vi "ziExample-Boxcar.vi"() -> ()   [LabVIEW 2009]
doc: "Control a Zurich instrument device via the LabOne Labview API. \nRequirements: Zurich Instruments UHFLI \nThis example retrives boxcar samples from a Zurich Instruments UHFLI instrument.\n\n© Zurich Instruments AG, www.zhinst.com"
uses:
  <instrlib>/Zurich Instruments LabOne/Public/Configure/ziSetValueDoubleArray.vi
  <instrlib>/Zurich Instruments LabOne/Public/Utility/ziTicksToS_single.vi
  <instrlib>/Zurich Instruments LabOne/Public/Configure/ziSetValueDouble.vi
  <instrlib>/Zurich Instruments LabOne/Public/Utility/ziTicksToS_vector.vi
  <instrlib>/Zurich Instruments LabOne/Public/Data/ziGetEventDoubleDataTS.vi
  <instrlib>/Zurich Instruments LabOne/Public/Data/ziGetEventPWAWave.vi
  <instrlib>/Zurich Instruments LabOne/Public/Data/ziGetEventIntDataTS.vi
  <instrlib>/Zurich Instruments LabOne/Zurich Instruments LabOne.lvlib
  <vilib>/Analysis/NI_AALBase.lvlib
panel:
  in  "boxcars/0/periods":dbl=1.0 caption="Boxcar Periods"
  in  "boxcars/0/windowsize":dbl=3e-09 caption="Window Size"
  in  "boxcars/0/windowstart":dbl=75.0 caption="Window Start"
  out "boxcarstd":dbl caption="Boxcar STD" format="%e"
  out "boxcaravg":dbl caption="Boxcar AVG" format="%e"
  out "periods":dbl caption="Periods" format="%0.2f"
  out "All Values (V) 2":cluster{"Timestamp(s)":dbl[], "Value":dbl[]}(graph)
  out "Error Out":errorcluster
  in  "Address":string="DEV"
  out "Selected Device":string
  out "Update Rate (1/s)":dbl(graph)
  out "All Values (V)":cluster{"Timestamp(s)":dbl[], "Value":dbl[]}(graph)
  in  "stop":bool
  # "ziExample-Boxcar.vi\nRequirements: UHFLI\nsee block diagram for VI description"
  # "Tested Devices:\n- UHFLI"
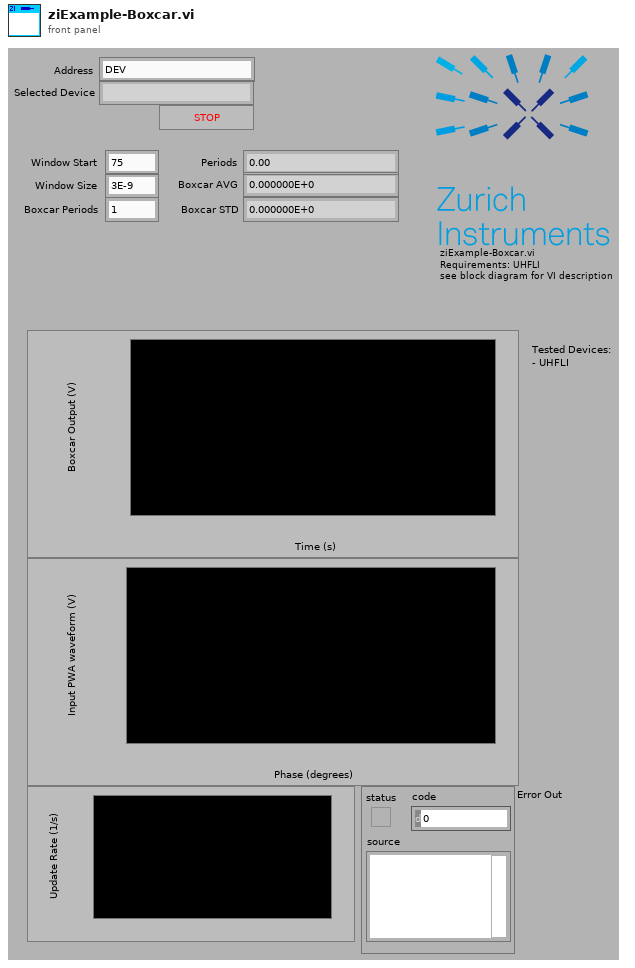
[diagram p1: front panel]
types:
  T1 = typedef "Zurich Instruments LabOne.lvlib/ziTypeHandle.ctl" = cluster{"handleValid":bool, "Conn":u64, "Path Prefix":string, "Handle":u64, "Connected":bool, "Clockbase(s)":dbl}
  T2 = typedef "Zurich Instruments LabOne.lvlib/ziTypeDoubleDataTS.ctl" = cluster{"Timestamp (ticks)":u64[], "Value":dbl[]}
  T3 = typedef "Zurich Instruments LabOne.lvlib/ziTypePWAWave.ctl" = cluster{"Timestamp (ticks)":u64, "SampleCount":u64, "InputSelect":i32, "OscSelect":i32, "Harmonic":i32, "BinCount":i32, "Frequency (Hz)":dbl, "PWAType":u8, "Mode":u8, "Overflow":u8, "Commensurable":u8, "BinPhase":dbl[], "X":dbl[], "Y":dbl[], "countBin":u32[]}
  T4 = typedef "Zurich Instruments LabOne.lvlib/ziTypeIntegerDataTS.ctl" = cluster{"Timestamp (ticks)":u64[], "Value":i64[]}
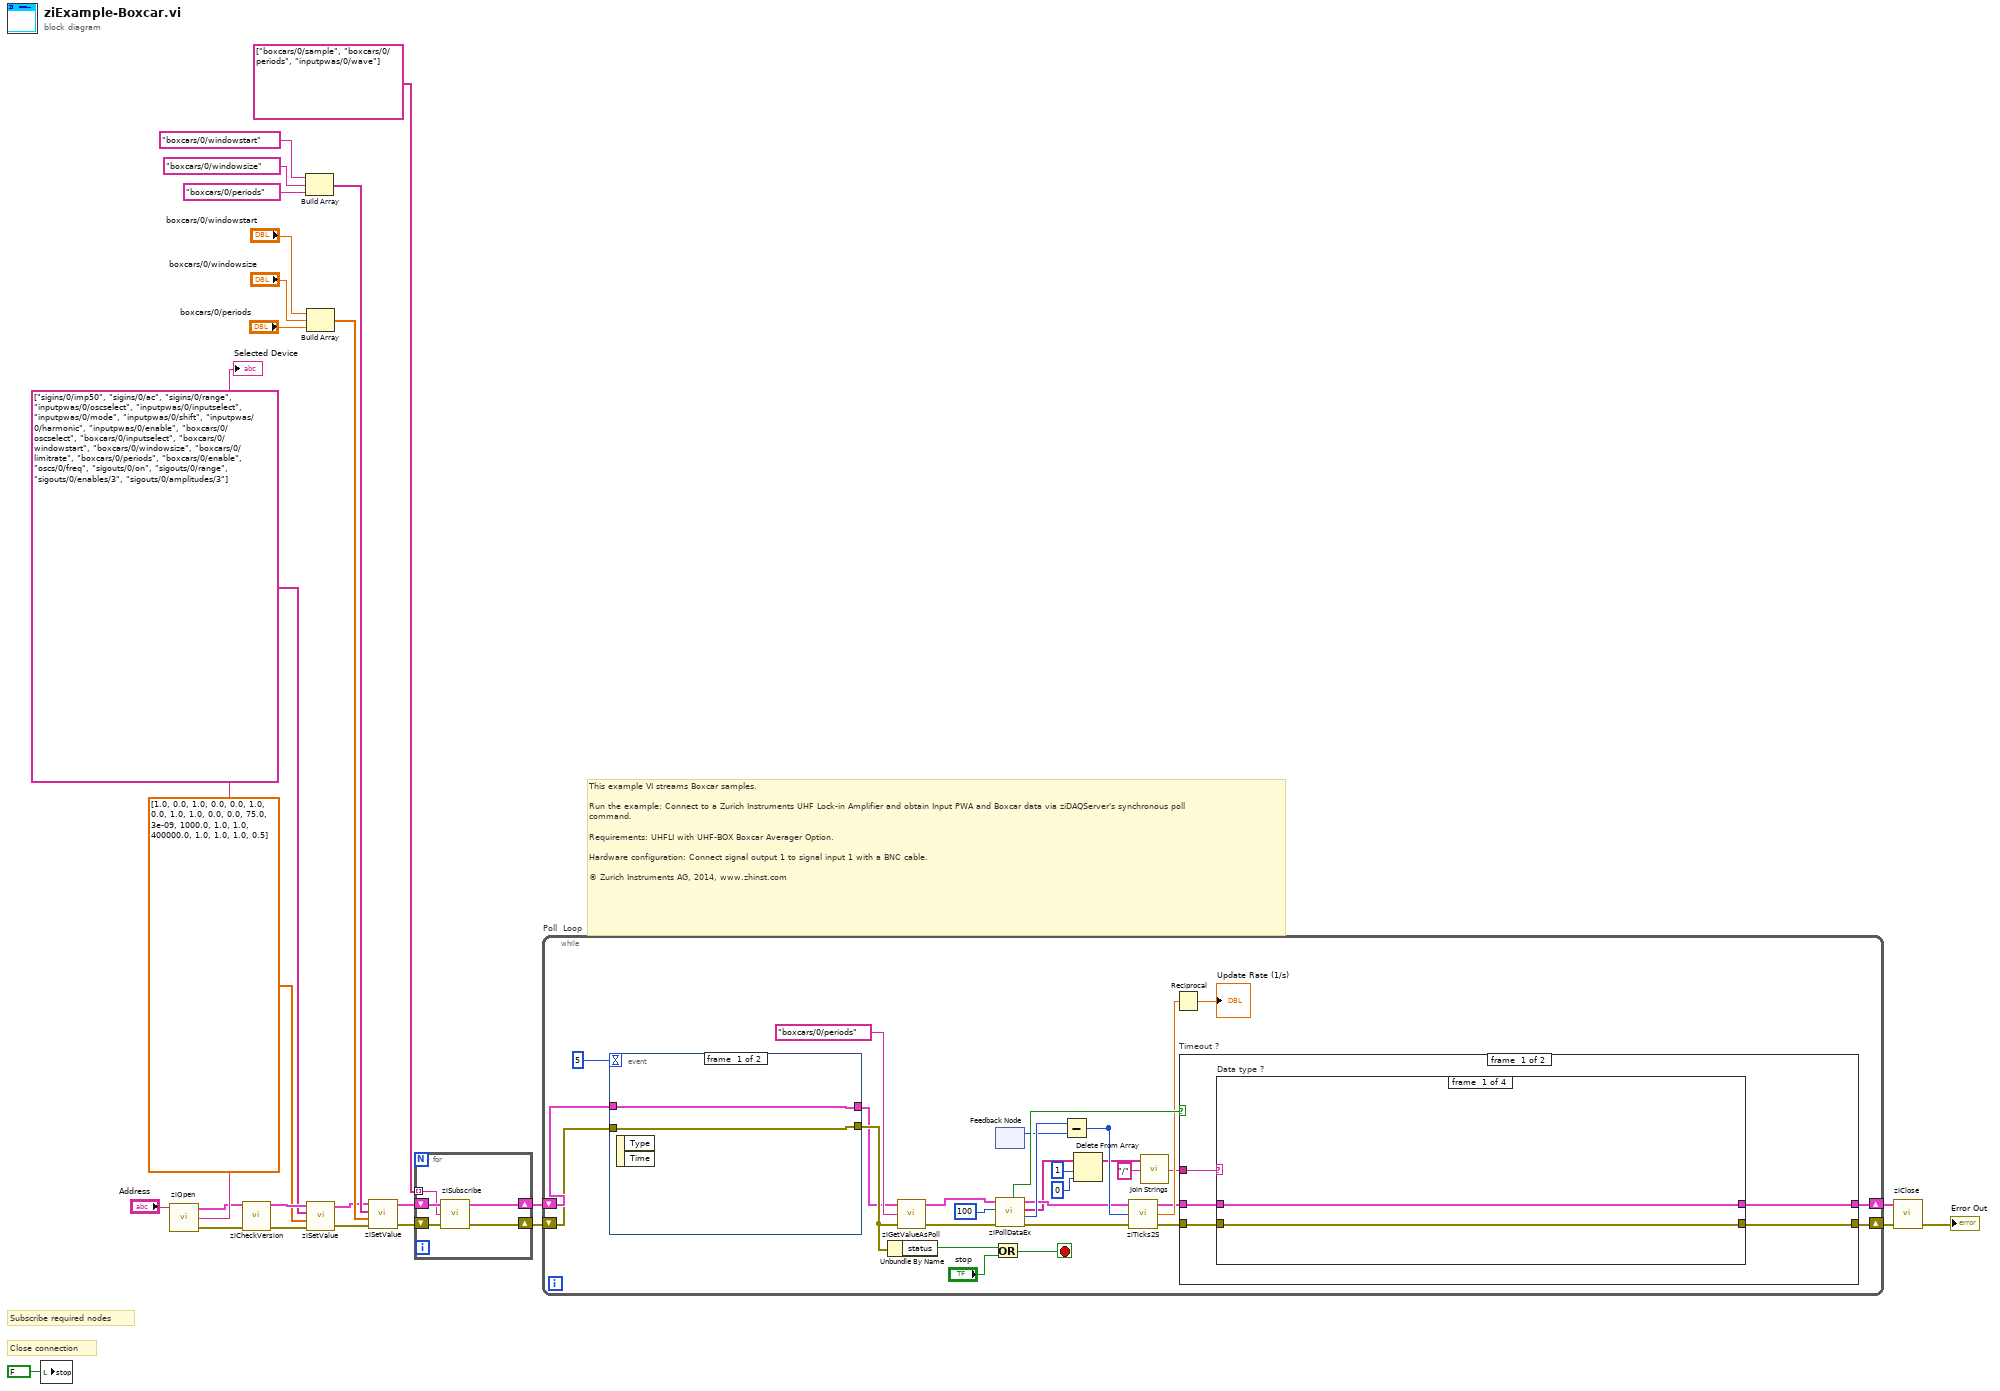
[diagram p0: block diagram]
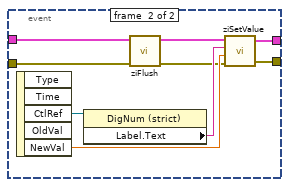
[diagram p2: hidden frame]
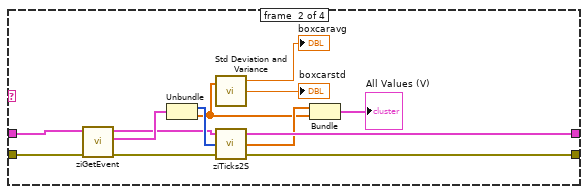
[diagram p3: hidden frame]
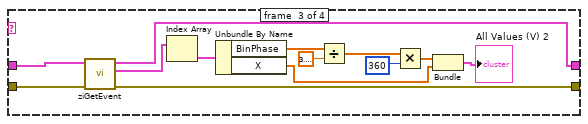
[diagram p4: hidden frame]
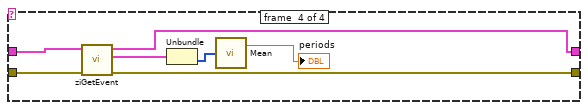
[diagram p5: hidden frame]
diagram:
  # "Close connection"
  # "Subscribe required nodes"
  # "This example VI streams Boxcar samples.\n\nRun the example: Connect to a Zurich Instruments UHF Lock-in Amplifier and obtain Input PWA and Boxcar data via ziDAQServer's synchronous poll command.\n\nRequirements: UHFLI with UHF-BOX Boxcar Averager Option.\n\nHardware configuration: Connect signal output 1 to signal input 1 with a BNC cable.\n\n© Zurich Instruments AG, 2014, www.zhinst.com"
  n1 = local write "stop"(FALSE ("Record")) -> ()
  n2 = call <instrlib>:"ziOpen.vi"("Address"="Address") -> ("Error Out"=w16:errorcluster, "Selected Device"=→"Selected Device":string, "HandleOut"=w19:T1)  [unwired: 1 in, 2 out]
  n3 = call <instrlib>:"ziCheckVersion.vi"("Handle In"=w19, "Error In"=w16) -> ("Handle Out"=w18:T1, "Error Out"=w17:errorcluster)  [unwired: 11 in, 1 out]
  n4 = Build Array("boxcars/0/windowstart" ("path"), "boxcars/0/windowsize" ("path"), "boxcars/0/periods" ("path")) -> (w6:string[])
  n5 = Build Array("boxcars/0/windowstart", "boxcars/0/windowsize", "boxcars/0/periods") -> (w5:dbl[])
  n6 = call-poly <instrlib>:"ziSetValue.vi"("Error In"=w17, "Values"=dbl[] [1.0, 0.0, 1.0, 0.0, 0.0, 1.0, 0.0, 1.0, 1.0, 0.0, 0.0, 75.0, 3e-09, 1000.0, 1.0, 1.0, 400000.0, 1.0, 1.0, 1.0, 0.5], "Paths"=string[] ["sigins/0/imp50", "sigins/0/ac", "sigins/0/range", "inputpwas/0/oscselect", "inputpwas/0/inputselect", "inputpwas/0/mode", "inputpwas/0/shift", "inputpwas/0/harmonic", "inputpwas/0/enable", "boxcars/0/oscselect", "boxcars/0/inputselect", "boxcars/0/windowstart", "boxcars/0/windowsize", "boxcars/0/limitrate", "boxcars/0/periods", "boxcars/0/enable", "oscs/0/freq", "sigouts/0/on", "sigouts/0/range", "sigouts/0/enables/3", "sigouts/0/amplitudes/3"], "Handle In"=w18) -> ("Error Out"=w1:errorcluster, "Handle Out"=w2:T1)  [unwired: 1 in]
  n7 = call-poly <instrlib>:"ziSetValue.vi"("Error In"=w1, "Values"=w5, "Paths"=w6, "Handle In"=w2) -> ("Error Out"=w3:errorcluster, "Handle Out"=w4:T1)  [unwired: 1 in]
  n8 = for {
    shift-right: [w32] -> w24
    shift-left: w4 -> [w30]
    shift-right: [w31] -> w23
    shift-left: w3 -> [w29]
    tunnel: string[] ["boxcars/0/sample", "boxcars/0/periods", "inputpwas/0/wave"] -> [w28] mode=indexing
    n9 = call <instrlib>:"ziSubscribe.vi"("error in"=w29, "Path ()"=w28, "Handle In"=w30) -> ("error out"=w31:errorcluster, "Handle Out"=w32:T1)  [unwired: 1 in]
  }
  n10 = while "Poll  Loop" {
    shift-right: [w60] -> w25
    shift-left: w24 -> [w36]
    shift-right: [w59] -> w26
    shift-left: w23 -> [w35]
    stop <- w56 stop-if-true
    n11 = event shown="[1] \"boxcars/0/windowstart\", \"boxcars/0/windowsize\", \"boxcars/0/periods\": Value Change" {
      selector: _ -> [_ _]
      dyn-events: _ -> [_ _]
      timeout: 5 -> [_ _]
      tunnel: w36 -> [w64 w68]
      tunnel: w35 -> [w63 w65]
      tunnel: [w64 w72] -> w33
      tunnel: [w63 w73] -> w34
      event #0 {
        n12 = event-data() -> ()  [unwired: 1 in, 2 out]
      }
      event #1 {
        n13 = event-data() -> ("CtlRef"=w71:refnum<vi>, "NewVal"=w69:dbl)  [unwired: 1 in, 3 out]
        n14 = property class="DigNum (strict)"(reference=w71) -> ("Label.Text"=w70:string)  [unwired: 1 in, 2 out]
        n15 = call <instrlib>:"ziFlush.vi"("error in"=w65, "Handle In"=w68) -> ("error out"=w66:errorcluster, "Handle Out"=w67:T1)  [unwired: 8 in]
        n16 = call-poly <instrlib>:"ziSetValue.vi"("Error In"=w66, "Value"=w69, "Path"=w70, "Handle In"=w67) -> ("Error Out"=w73:errorcluster, "Handle Out"=w72:T1)  [unwired: 1 in]
      }
    }
    n17 = Unbundle By Name(w34) -> ("status"=w58:bool)
    n18 = call <instrlib>:"ziGetValueAsPoll.vi"("error in"=w34, "Path"="boxcars/0/periods", "Handle in"=w33) -> ("error out"=w39:errorcluster, "Handle out"=w38:T1)  [unwired: 1 in]
    n19 = Or(x=w58, y="stop") -> (x .or. y?=w56:bool)
    n20 = feedback #1() -> (w52:u64)  [unwired: 1 in]
    n21 = call <instrlib>:"ziPollDataEx.vi"("error in"=w39, "Timeout ms (50)"=100 ("TimeOut ms (50)"), "Handle In"=w38) -> ("error out"=w48:errorcluster, "Timestamp (ticks)"=w53:u64, "PathArray"=w42:string[], "Handle Out"=w50:T1, "Timed Out"=w61:bool)  [unwired: 1 in, 3 out]
    n22 = Subtract(x=w53, y=w52) -> (x-y=w51:u64)
    n23 = Delete From Array(array=w42, length=1, index=0) -> (array with subset deleted=w41:string[])  [unwired: 1 out]
    n24 = call-poly <instrlib>:"ziTicks2S.vi"("Error In"=w48, "Timestamp(ticks)"=w51, "Handle In"=w50) -> ("Error Out"=w47:errorcluster, "Timestamp(s)"=w55:dbl, "Handle Out"=w49:T1)
    n25 = call <vilib>:"Join Strings.vi"("Separator (,)"="/", "Strings In"=w41) -> ("String"=w45:string)  [unwired: 1 in]
    n26 = Reciprocal(x=w55) -> (1/x=→"Update Rate (1/s)":dbl)
    n27 = case "Timeout ?" shown="False" w61 {
      tunnel: w49 -> [w78 w115]
      tunnel: [w77 w115] -> w60
      tunnel: w47 -> [w76 w114]
      tunnel: [w75 w114] -> w59
      tunnel: w45 -> [w74 _]
      frame #0 {
        n28 = case "Data type ?" shown="\"inputpwas/0/wave\"" w74 {
          tunnel: w78 -> [w80 w85 w105 w111]
          tunnel: [w80 w90 w102 w110] -> w77
          tunnel: w76 -> [w79 w86 w106 w112]
          tunnel: [w79 w87 w101 w109] -> w75
          frame #0 {
          }
          frame #1 {
            n29 = call-poly <instrlib>:"ziGetEvent.vi"("Error In"=w86, "Handle In"=w85) -> ("Error Out"=w89:errorcluster, "Sample Out"=w93:T2, "Handle Out"=w88:T1)  [unwired: 7 in]
            n30 = Unbundle(w93) -> ("Timestamp (ticks)"=w91:u64[], "Value"=w83:dbl[])
            n31 = call <vilib>:"Std Deviation and Variance.vi"("X"=w83) -> ("mean"=→"boxcaravg":dbl, "standard deviation"=→"boxcarstd":dbl)  [unwired: 1 in, 1 out]
            n32 = call-poly <instrlib>:"ziTicks2S.vi"("Error In"=w89, "Timestamp (ticks)"=w91, "Handle In"=w88) -> ("Error Out"=w87:errorcluster, "Timestamp(s)"=w84:dbl[], "Handle Out"=w90:T1)
            n33 = Bundle("Timestamp(s)"=w84, "Value"=w83) -> (→"All Values (V)":cluster{"Timestamp(s)":dbl[], "Value":dbl[]})  [unwired: 1 in]
          }
          frame #2 {
            n34 = call-poly <instrlib>:"ziGetEvent.vi"("Error In"=w106, "Handle In"=w105) -> ("Error Out"=w101:errorcluster, "PWAWaves Out"=w104:T3[], "Handle Out"=w102:T1)  [unwired: 7 in]
            n35 = Index Array(array=w104) -> (element=w103:T3)  [unwired: 1 in]
            n36 = Unbundle By Name(w103) -> ("BinPhase"=w97:dbl[], "X"=w100:dbl[])
            n37 = Divide(x=w97, y=3.141592653589793) -> (x/y=w96:dbl[])
            n38 = Multiply(x=w96, y=360) -> (x*y=w94:dbl[])
            n39 = Bundle(w94, "X"=w100) -> (→"All Values (V) 2":cluster{dbl[], "X":dbl[]})  [unwired: 1 in]
          }
          frame #3 {
            n40 = call-poly <instrlib>:"ziGetEvent.vi"("Error In"=w112, "Handle In"=w111) -> ("Error Out"=w109:errorcluster, "Sample Out"=w113:T4, "Handle Out"=w110:T1)  [unwired: 7 in]
            n41 = Unbundle(w113) -> ("Value"=w108:i64[])  [unwired: 1 out]
            n42 = call <vilib>:"Mean.vi"("X"=w108) -> ("mean"=→"periods":dbl)  [unwired: 1 out]
          }
        }
      }
      frame #1 {
        # "Timeout, no action."
      }
    }
  }
  n43 = call <instrlib>:"ziClose.vi"("Error In"=w26, "Handle In"=w25) -> ("Error Out"=→"Error Out":errorcluster)  [unwired: 3 out]
